vi "Helper - UTM Location to Log String.vi"(9 "Input":T1 {"North" format="%#_10f"; "East" format="%#_8f"}, 10 "Selector":string, 11 "PrevString":string) -> (3 "Output":string)   [LabVIEW 2011]
doc: "Part of Helper - Data to String.vi. Look there for more details."
uses:
  2 Typedefs/UTM Location.ctl
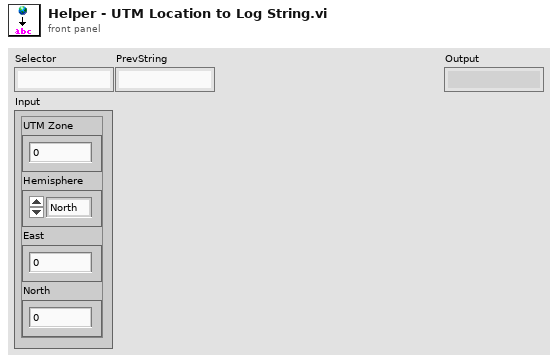
[diagram p1: front panel]
types:
  T1 = typedef "UTM Location.ctl" = cluster{"UTM Zone":dbl, "Hemisphere":enum16{"North", "South"}, "East":dbl, "North":dbl}
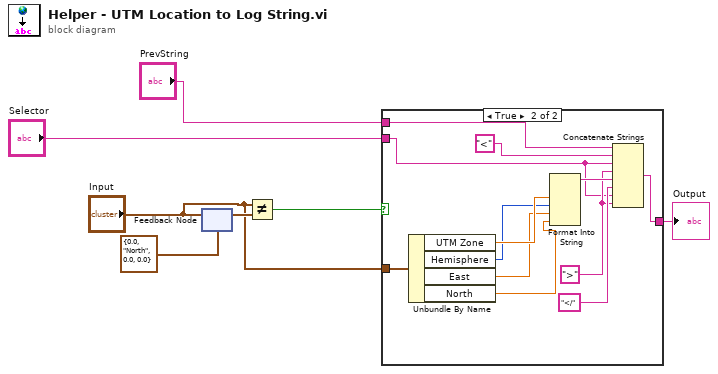
[diagram p0: block diagram]
diagram:
  n1 = feedback #1(T1 {"UTM Zone"=0.0, "Hemisphere"=enum."North", "East"=0.0, "North"=0.0} ("Robot UTM Location")) -> (w4:T1)
  n2 = feedback-in #1("Input") -> ()
  n3 = Not Equal?(x="Input", y=w4) -> (x != y?=w1:bool)
  n4 = case shown="True" w1 {
    tunnel: [w8 w20] -> w6
    tunnel: "Selector" -> [_ w9]
    tunnel: "Input" -> [_ w15]
    tunnel: "PrevString" -> [w8 w10]
    frame False {
    }
    frame True {
      w16 = ">" ("string")
      n5 = Unbundle By Name(w15) -> ("UTM Zone"=w14:dbl, "Hemisphere"=w13:enum16{"North", "South"}, "East"=w12:dbl, "North"=w11:dbl)
      n6 = Format Into String(w14, w13, w12, w11) -> (resulting string=w19:string)  [unwired: 3 in, 1 out]
      n7 = Concatenate Strings(w10, "<" ("string"), w9, w16, w19, "</" ("string"), w9, w16) -> (w20:string)
    }
  }
  "Output" <- w6
